vi "Tab Control Ref.vi"(8 "error out":errorcluster, 9 "Label Text":string, 10 "Array In":string[](array[string]), 11 "TabControl Reference":refnum<vi>) -> (2 "Array Out":string[](array[string]), 3 "ControlsOnPage":refnum<vi>[](array[refnum]))   [LabVIEW 2021]
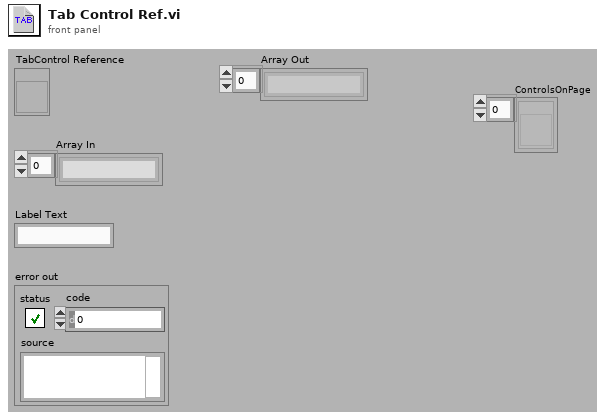
[diagram p1: front panel]
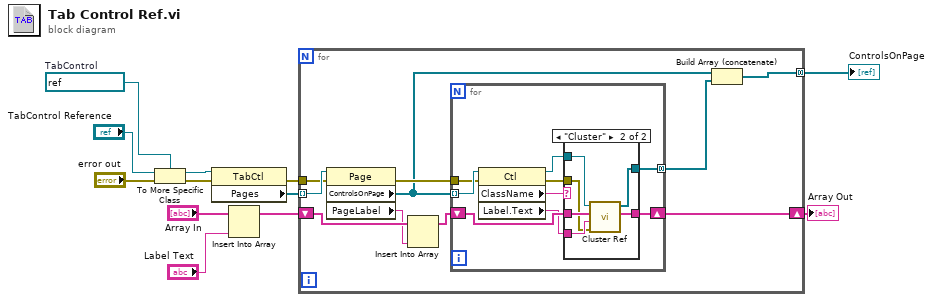
[diagram p0: block diagram]
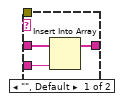
[diagram p2: hidden frame]
diagram:
  w6 = refnum<vi> refnum  # TabControl
  n1 = To More Specific Class(target class=w6, reference="TabControl Reference", error in="error out") -> (specific class reference=w4:refnum<vi>, error out=w2:errorcluster)
  n2 = property class="TabCtl"(reference=w4, error in=w2) -> (error out=w11:errorcluster, "Pages"=w7:refnum<vi>[])  [unwired: 1 out]
  n3 = Insert Into Array(array="Array In", new element="Label Text") -> (w9:string[])  [unwired: 1 in]
  n4 = for {
    tunnel: w7 -> [w22] mode=indexing
    shift-right: [w21] -> w10
    shift-left: w9 -> [w20]
    tunnel: w11 -> [w17]
    tunnel: [w14] -> w1 mode=concatenating
    n5 = property class="Page"(reference=w22, error in=w17) -> (error out=w16:errorcluster, "ControlsOnPage"=w15:refnum<vi>[], "PageLabel"=w18:string)  [unwired: 1 out]
    n6 = Insert Into Array(array=w20, new element=w18) -> (w19:string[])  [unwired: 1 in]
    n7 = for {
      tunnel: w15 -> [w29] mode=indexing
      shift-right: [w30] -> w21
      shift-left: w19 -> [w31]
      tunnel: w16 -> [w28]
      tunnel: [w23] -> w13 mode=concatenating
      n8 = property class="Ctl"(reference=w29, error in=w28) -> (reference out=w25:refnum<vi>, error out=w24:errorcluster, "ClassName"=w27:string, "Label.Text"=w26:string)
      n9 = case shown="\"Cluster\"" w27 {
        tunnel: w31 -> [w34 w40]
        tunnel: [w32 w36] -> w30
        tunnel: w26 -> [w33 w38]
        tunnel: w25 -> [_ w39]
        tunnel: w24 -> [_ w37]
        tunnel: [_ w35] -> w23
        frame "", Default {
          n10 = Insert Into Array(array=w34, new element=w33) -> (w32:string[])  [unwired: 1 in]
        }
        frame "Cluster" {
          n11 = call "Cluster Ref.vi"("error out"=w37, "Label Text"=w38, "Input Array"=w40, "Cluster Reference"=w39) -> ("Array Out"=w36:string[], "Controls[]"=w35:refnum<vi>[])  [unwired: 6 in]
        }
      }
    }
    n12 = Build Array (concatenate)(w15, w13) -> (w14:refnum<vi>[])
  }
  "Array Out" <- w10
  "ControlsOnPage" <- w1
